vi "Check Deadline.vi"(8 "error in (no error)":errorcluster, 11 "Timer in":refnum<class "Timer.lvclass">) -> (0 "error out":errorcluster, 3 "Timer out":refnum<class "Timer.lvclass">)   [LabVIEW 2023, in "Timer.lvlib" / "Timer.lvclass"]
uses:
  Timer.lvclass
  Timer.lvclass/Timer.ctl
  <vilib>/ActorFramework/Actor/Actor.lvclass/Actor.ctl
  <vilib>/ActorFramework/Message Enqueuer/Message Enqueuer.lvclass/Message Enqueuer.ctl
  Application Messages/Automation_TaskCompleted Msg/Automation_TaskCompleted Msg.lvclass/Automation_TaskCompleted Msg.ctl
  <vilib>/ActorFramework/Message Enqueuer/Init from Existing Queue.vi
  <vilib>/ActorFramework/Message Enqueuer/Enqueue.vi
  Timer Messages/Check Deadline Msg/Check Deadline Msg.lvclass
  Application Messages/Automation_TaskCompleted Msg/Automation_TaskCompleted Msg.lvclass
  <vilib>/ActorFramework/Message Priority Queue/Priority Enqueue.vi
  <vilib>/ActorFramework/Message Enqueuer/Message Enqueuer.lvclass
  <vilib>/ActorFramework/Actor/Actor.lvclass
  C:/Program Files/National Instruments/LabVIEW 2023/vi.lib/ActorFramework/Actor/Actor.lvclass
  C:/FLASH/Development/Timer/Timer.lvclass
panel:
  out "output cluster":cluster{"Progress":u8, "Time Remaining (s)":dbl}
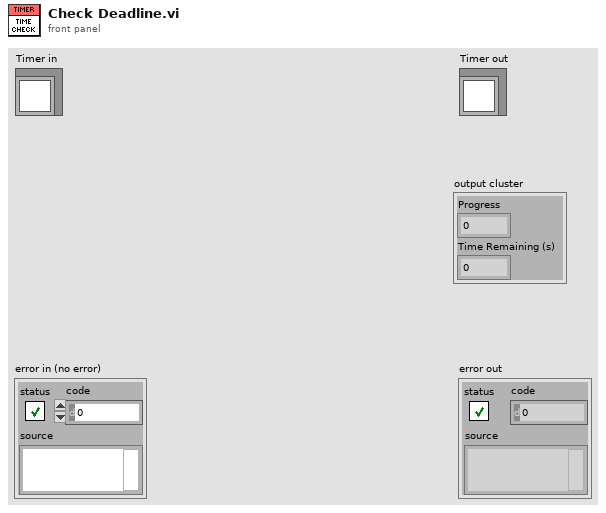
[diagram p1: front panel]
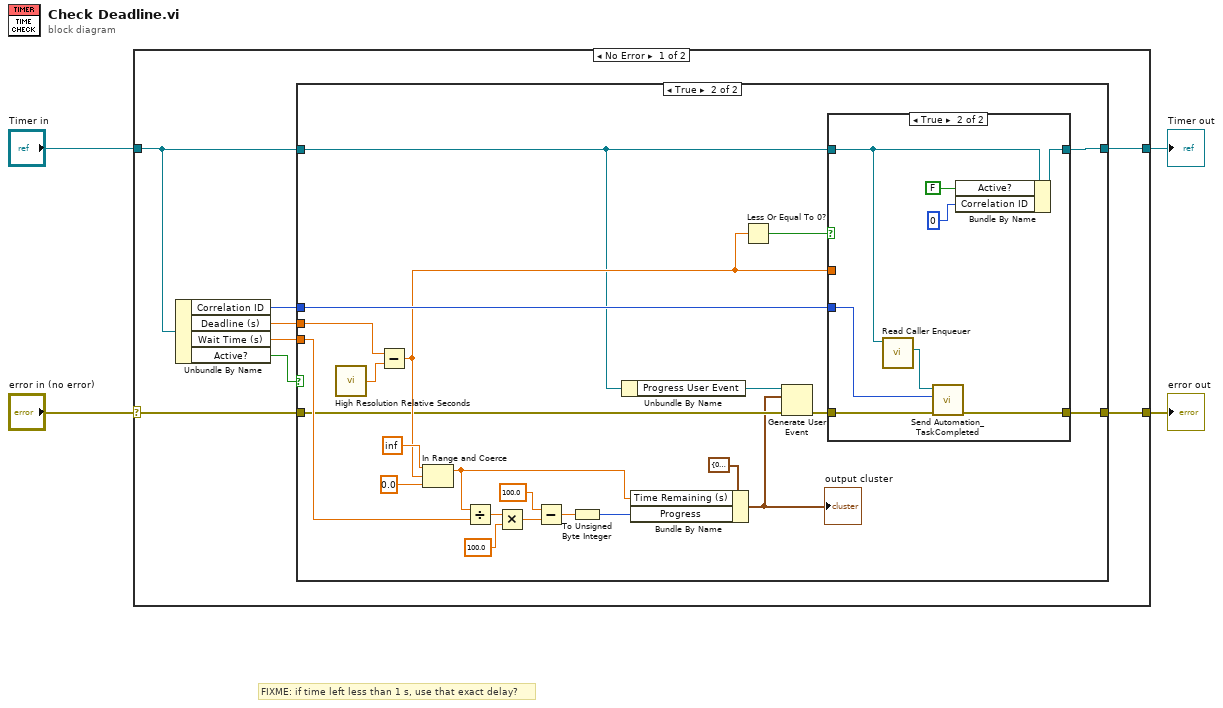
[diagram p0: block diagram]
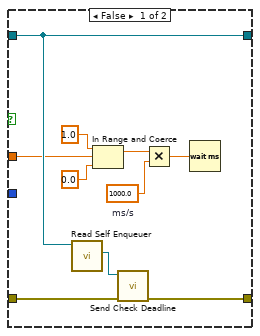
[diagram p3: hidden frame]
diagram:
  # "FIXME: if time left less than 1 s, use that exact delay?"
  n1 = case shown="No Error" "error in (no error)" {
    selector: "error in (no error)" -> [w12 w57]
    tunnel: [w9 w57] -> w3
    tunnel: [w6 w56] -> w1
    tunnel: "Timer in" -> [w7 w56]
    frame No Error {
      n2 = Unbundle By Name(w7) -> ("Correlation ID"=w11:u32, "Deadline (s)"=w10:dbl, "Wait Time (s)"=w8:dbl, "Active?"=w5:bool)
      n3 = case shown="True" w5 {
        tunnel: w12 -> [w13 w18]
        tunnel: w11 -> [_ w37]
        tunnel: w10 -> [_ w36]
        tunnel: [w13 w21] -> w9
        tunnel: w8 -> [_ w26]
        tunnel: w7 -> [w14 w15]
        tunnel: [w14 w22] -> w6
        frame False {
          # "Timer aborted early"
        }
        frame True {
          n4 = call <vilib>:"High Resolution Relative Seconds.vi"() -> ("relative seconds"=w35:dbl)
          n5 = Subtract(x=w36, y=w35) -> (x-y=w20:dbl)
          n6 = In Range and Coerce(upper limit=inf, x=w20, lower limit=0.0) -> (coerced(x)=w25:dbl)  [unwired: 1 out]
          n7 = Divide(x=w25, y=w26) -> (x/y=w33:dbl)
          n8 = Multiply(x=w33, y=100.0) -> (x*y=w31:dbl)
          n9 = Subtract(x=100.0, y=w31) -> (x-y=w28:dbl)
          n10 = To Unsigned Byte Integer(number=w28) -> (unsigned 8bit integer=w27:u8)
          n11 = Unbundle By Name(w15) -> ("Progress User Event"=w19:refnum<user-event>)
          n12 = Bundle By Name(cluster=cluster{"Progress":u8, "Time Remaining (s)":dbl} {"Progress"=0, "Time Remaining (s)"=0.0}, "Time Remaining (s)"=w25, "Progress"=w27) -> (w16:cluster{"Progress":u8, "Time Remaining (s)":dbl})
          "output cluster" <- w16
          n13 = Less Or Equal To 0?(x=w20) -> (x <= 0?=w34:bool)
          n14 = Generate User Event(user event=w19, event data cluster=w16, error in=w18) -> (error out=w17:errorcluster)  [unwired: 1 in, 1 out]
          n15 = case shown="True" w34 {
            tunnel: w17 -> [w47 w55]
            tunnel: [w46 w54] -> w21
            tunnel: w37 -> [_ w53]
            tunnel: w15 -> [w44 w51]
            tunnel: [w44 w50] -> w22
            tunnel: w20 -> [w41 _]
            frame False {
              w38 = 1000.0  # ms/s
              n16 = call <vilib>:"Read Self Enqueuer.vi"("Actor"=w44) -> ("Self Enqueuer"=w45:refnum<class "Message Enqueuer.lvclass">)  [unwired: 10 in]
              n17 = In Range and Coerce(upper limit=1.0 ("milliseconds to wait"), x=w41, lower limit=0.0 ("milliseconds to wait")) -> (coerced(x)=w40:dbl)  [unwired: 1 out]
              n18 = call "Send Check Deadline.vi"("error in (no error)"=w47, "Message Enqueuer"=w45) -> ("error out"=w46:errorcluster)  [unwired: 8 in, 1 out]
              n19 = Multiply(x=w40, y=w38) -> (x*y=w39:dbl)
              n20 = Wait (ms)(milliseconds to wait=w39) -> ()  [unwired: 1 out]
            }
            frame True {
              n21 = call <vilib>:"Read Caller Enqueuer.vi"("Actor"=w51) -> ("Caller Enqueuer"=w52:refnum<class "Message Enqueuer.lvclass">)  [unwired: 10 in]
              n22 = call "Send Automation_TaskCompleted.vi"("error in (no error)"=w55, "Correlation ID"=w53, "Message Enqueuer"=w52) -> ("error out"=w54:errorcluster)  [unwired: 7 in, 1 out]
              n23 = Bundle By Name(cluster=w51, "Active?"=FALSE, "Correlation ID"=u32 0) -> (w50:refnum<class "Timer.lvclass">)
            }
          }
        }
      }
    }
    frame Error {
    }
  }
  "error out" <- w3
  "Timer out" <- w1
